vi "action.vi"(0 "HGF_FGV_VisitSubset":refnum<class "HGF_FGV_VisitSubSet.lvclass">, 2 "Objects":refnum<class>[](array[class]), 5 "error in (no error)":errorcluster) -> (14 "dup HGF_FGV_VisitSubset":refnum<class "HGF_FGV_VisitSubSet.lvclass">, 16 "dup Objects":refnum<class>[](array[class]), 19 "error out":errorcluster)   [LabVIEW 2012, in "HGF_FGV.lvlib" / "HGF_FGV_VisitSubSet.lvclass"]
doc: "Apply Visitors action to subset of objects in FGV instance."
uses:
  HGF_FGV_VisitSubSet.lvclass
  HGF_Visitable/HGF_Visitable.lvclass
  HGF_FGV_VisitSubSet.lvclass/HGF_FGV_VisitSubSet.ctl
  HGF_FGV_Visitor/HGF_FGV_Visitor.lvclass
  HGF_Visitor/HGF_Visitor.lvclass
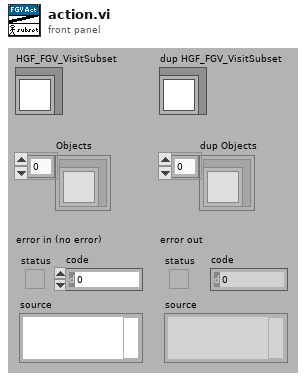
[diagram p1: front panel]
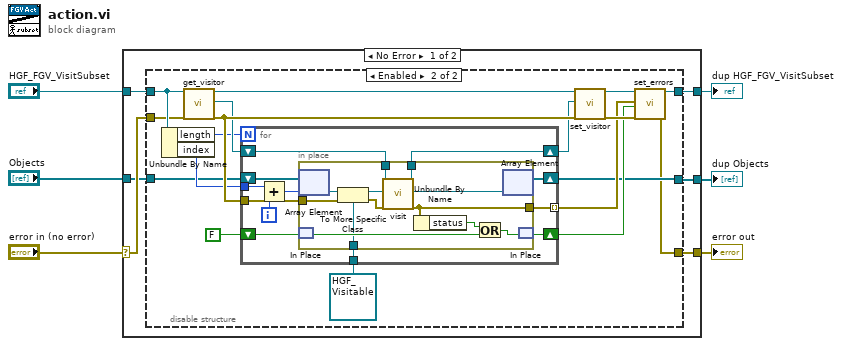
[diagram p0: block diagram]
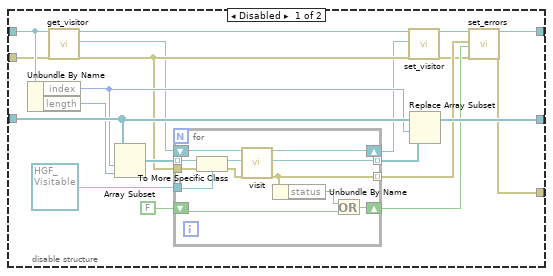
[diagram p2: hidden frame]
diagram:
  n1 = case shown="No Error" "error in (no error)" {
    selector: "error in (no error)" -> [w11 w89]
    tunnel: [w7 w89] -> w6
    tunnel: [w8 w88] -> w5
    tunnel: "HGF_FGV_VisitSubset" -> [w12 w88]
    tunnel: [w9 w87] -> w4
    tunnel: "Objects" -> [w10 w87]
    frame No Error {
      n2 = disable-structure shown="Enabled" {
        disable-tunnel: w12 -> [w32 w50]
        disable-tunnel: w11 -> [w30 w49]
        disable-tunnel: w10 -> [w29 w48]
        disable-tunnel: [w28 w46] -> w9
        disable-tunnel: [w17 w47] -> w8
        disable-tunnel: [w13 w45] -> w7
        frame Disabled {
          n3 = Unbundle By Name(w32) -> ("index"=w27:u32, "length"=w26:i32)
          n4 = call "get_visitor.vi"("HGF_FGV_Visitor"=w32, "error in (no error)"=w30) -> ("dup HGF_FGV_Visitor"=w31:refnum<class "HGF_FGV_VisitSubSet.lvclass">, "visitor"=w21:refnum<class "HGF_Visitor.lvclass">, "error out"=w23:errorcluster)  [unwired: 15 in]
          n5 = Array Subset(array=w29, index=w27, length=w26) -> (w25:refnum<class>[])
          n6 = for {
            tunnel: w25 -> [w43] mode=indexing
            tunnel: refnum<class "HGF_Visitable.lvclass"> refnum ("HGF_Visitable.lvclass") -> [w41]
            tunnel: [w39] -> w22 mode=indexing
            shift-right: [w37] -> w20
            shift-left: w21 -> [w38]
            tunnel: w23 -> [w40]
            tunnel: [w36] -> w16 mode=indexing
            shift-right: [w35] -> w15
            shift-left: FALSE -> [w33]
            n7 = To More Specific Class(target class=w41, reference=w43, error in=w40) -> (specific class reference=w42:refnum<class "HGF_Visitable.lvclass">, error out=w44:errorcluster)
            n8 = call "visit.vi"("HGF_Visitor"=w38, "HGF_Visitable"=w42, "error in (no error)"=w44) -> ("dup HGF_Visitor"=w37:refnum<class "HGF_Visitor.lvclass">, "dup HGF_Visitable"=w39:refnum<class "HGF_Visitable.lvclass">, "error out"=w36:errorcluster)  [unwired: 14 in]
            n9 = Unbundle By Name(w36) -> ("status"=w34:bool)
            n10 = Or(x=w34, y=w33) -> (x .or. y?=w35:bool)
          }
          n11 = call "set_visitor.vi"("HGF_FGV_Visitor"=w31, "visitor"=w20, "error in (no error)"=w23) -> ("dup HGF_FGV_Visitor"=w18:refnum<class "HGF_FGV_VisitSubSet.lvclass">, "error out"=w14:errorcluster)  [unwired: 15 in]
          n12 = Replace Array Subset(array=w29, new element=w22, index=w27) -> (w28:refnum<class>[])
          n13 = call "set_errors.vi"("HGF_FGV_Visitor"=w18, "Errors"=w16, "error"=w15, "error in (no error)"=w14) -> ("dup HGF_FGV_Visitor"=w17:refnum<class "HGF_FGV_VisitSubSet.lvclass">, "error out"=w13:errorcluster)  [unwired: 14 in]
        }
        frame Enabled {
          n14 = Unbundle By Name(w50) -> ("length"=w51:i32, "index"=w52:u32)
          n15 = call "get_visitor.vi"("HGF_FGV_Visitor"=w50, "error in (no error)"=w49) -> ("dup HGF_FGV_Visitor"=w56:refnum<class "HGF_FGV_VisitSubSet.lvclass">, "visitor"=w53:refnum<class "HGF_Visitor.lvclass">, "error out"=w58:errorcluster)  [unwired: 15 out]
          n16 = for {
            N: w51 -> [_]
            shift-right: [w73] -> w46
            shift-left: w48 -> [w74]
            tunnel: w52 -> [w72]
            shift-right: [w68] -> w57
            shift-left: w53 -> [w69]
            tunnel: [w66] -> w59 mode=indexing
            tunnel: w58 -> [w65]
            shift-right: [w64] -> w60
            shift-left: FALSE -> [w67]
            tunnel: refnum<class "HGF_Visitable.lvclass"> refnum ("HGF_Visitable.lvclass") -> [w63]
            i -> [w71]
            n17 = Add(x=w72, y=w71) -> (x+y=w70:u32)
            n18 = in-place {
              in-place-border: w69 -> [w81]
              in-place-border: [w80] -> w68
              in-place-border: [w77] -> w66
              in-place-border: w65 -> [w76]
              in-place-border: w63 -> [w75]
              n19 = in-place-array #1(w74, w70) -> (w83:refnum<class>)
              n20 = in-place-match #2(w67) -> (w79:bool)
              n21 = To More Specific Class(target class=w75, reference=w83, error in=w76) -> (specific class reference=w85:refnum<class "HGF_Visitable.lvclass">, error out=w84:errorcluster)
              n22 = call "visit.vi"("HGF_Visitor"=w81, "HGF_Visitable"=w85, "error in (no error)"=w84) -> ("dup HGF_Visitor"=w80:refnum<class "HGF_Visitor.lvclass">, "dup HGF_Visitable"=w82:refnum<class "HGF_Visitable.lvclass">, "error out"=w77:errorcluster)  [unwired: 14 out]
              n23 = Unbundle By Name(w77) -> ("status"=w86:bool)
              n24 = Or(x=w86, y=w79) -> (x .or. y?=w78:bool)
              n25 = in-place-array #1(w82) -> (w73:refnum<class>[])  [unwired: 1 out]
              n26 = in-place-match #2(w78) -> (w64:bool)
            }
          }
          n27 = call "set_visitor.vi"("HGF_FGV_Visitor"=w56, "visitor"=w57, "error in (no error)"=w58) -> ("dup HGF_FGV_Visitor"=w55:refnum<class "HGF_FGV_VisitSubSet.lvclass">, "error out"=w61:errorcluster)  [unwired: 15 out]
          n28 = call "set_errors.vi"("HGF_FGV_Visitor"=w55, "Errors"=w59, "error"=w60, "error in (no error)"=w61) -> ("dup HGF_FGV_Visitor"=w47:refnum<class "HGF_FGV_VisitSubSet.lvclass">, "error out"=w45:errorcluster)  [unwired: 14 out]
        }
      }
    }
    frame Error {
    }
  }
  "error out" <- w6
  "dup HGF_FGV_VisitSubset" <- w5
  "dup Objects" <- w4
